vi "窗格_所有窗格居中显示.vi"(8 "error in (no error)":errorcluster caption="错误输入（无错误）") -> (0 "error out":errorcluster caption="错误输出")   [LabVIEW 2018]
uses:
  <vilib>/Utility/miscctls.llb/LVPointTypeDef.ctl
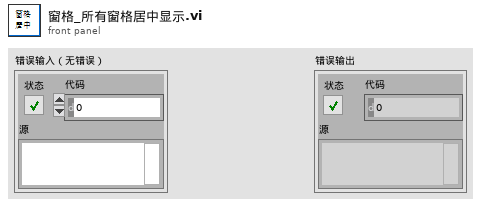
[diagram p1: front panel]
types:
  T1 = typedef "LVPointTypeDef.ctl" = cluster{"Horizontal":i16, "Vertical":i16}
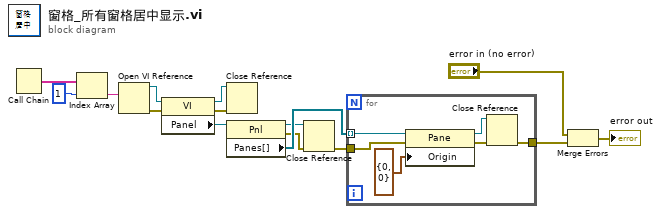
[diagram p0: block diagram]
diagram:
  n1 = Call Chain() -> (call chain=w12:string[])
  n2 = Index Array(array=w12, index=1 ("索引")) -> (element=w10:string)
  n3 = Open VI Reference(vi path=w10) -> (vi reference=w9:refnum<vi>, error out=w8:errorcluster)  [unwired: 5 in]
  n4 = property on="属性节点" class="VI"(reference=w9, error in=w8) -> (reference out=w4:refnum<vi>, error out=w5:errorcluster, "Panel"=w3:refnum<vi>)
  n5 = Close Reference(reference=w4, error in (no error)=w5) -> ()  [unwired: 1 out]
  n6 = property on="属性节点" class="Pnl"(reference=w3) -> (reference out=w6:refnum<vi>, error out=w7:errorcluster, "Panes[]"=w13:refnum<vi>[])  [unwired: 1 in]
  n7 = Close Reference(reference=w6, error in (no error)=w7) -> (error out=w2:errorcluster)
  n8 = for {
    tunnel: w13 -> [w21] mode=indexing
    tunnel: [w17] -> w1
    tunnel: w2 -> [w16]
    n9 = property on="属性节点" class="Pane"(reference=w21, error in=w16, "Origin"=T1 {"Horizontal"=0, "Vertical"=0} ("原点")) -> (reference out=w18:refnum<vi>, error out=w19:errorcluster)
    n10 = Close Reference(reference=w18, error in (no error)=w19) -> (error out=w17:errorcluster)
  }
  n11 = Merge Errors("error in (no error)", w1) -> (→"error out":errorcluster)
